vi "Stop Editor.vi"(8 "error in (no error)":errorcluster, 11 "Editor Handler in":refnum<class "Image Editor Handler.lvclass">) -> (0 "error out":errorcluster, 3 "Editor Handler out":refnum<class "Image Editor Handler.lvclass">)   [LabVIEW 2017, in "LV Image Editor Framework.lvlib" / "Image Editor Handler.lvclass"]
uses:
  Image Editor Handler.lvclass
  Image Editor Handler.lvclass/Image Editor Handler.ctl
  Forms/Shape/Shape.lvclass
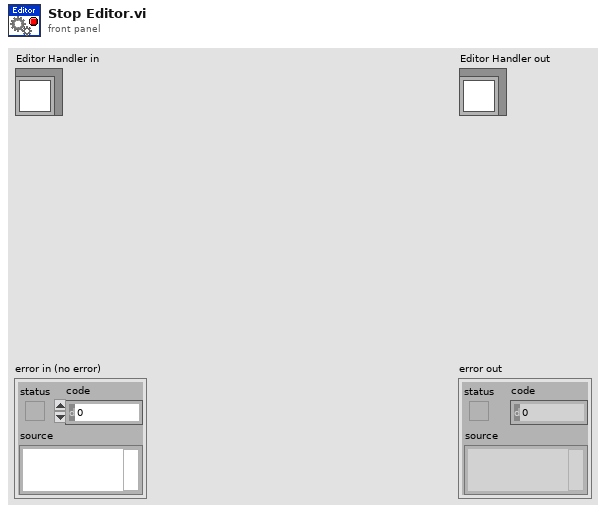
[diagram p1: front panel]
types:
  T1 = typedef "LV Image Editor Framework.lvlib/Image Editor Handler.lvclass/Editor Events.ctl" = cluster{"Stop":refnum<user-event>, "Image Events":cluster{"AddShape":refnum<user-event>, "Paint":refnum<user-event>, "RemoveShape":refnum<user-event>, "RefreshShape ByRef":refnum<user-event>, "ShapePropertyChange":refnum<user-event>, "RemoveShape ByRef":refnum<user-event>}, "RequestShapes":refnum<user-event>, "Custom":refnum<user-event>}
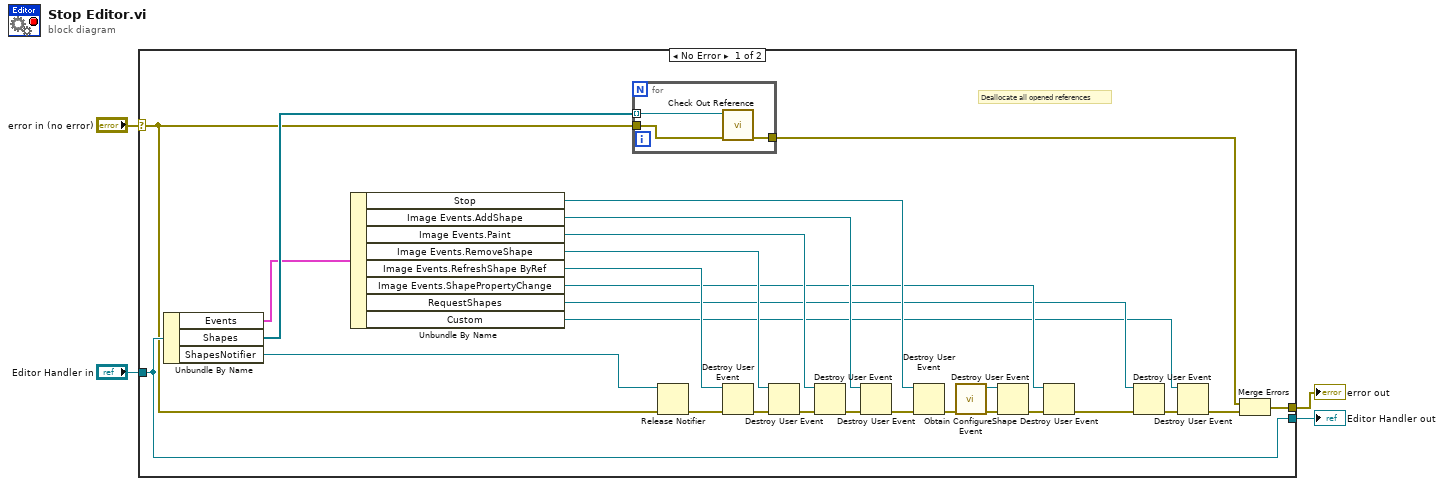
[diagram p0: block diagram]
diagram:
  n1 = case shown="No Error" "error in (no error)" {
    selector: "error in (no error)" -> [w7 w36]
    tunnel: [w17 w36] -> w3
    tunnel: [w31 w35] -> w1
    tunnel: "Editor Handler in" -> [w31 w35]
    frame No Error {
      # "Deallocate all opened references"
      n2 = Unbundle By Name(w31) -> ("Events"=w29:T1, "Shapes"=w30:refnum<data-value>[], "ShapesNotifier"=w13:refnum<notifier>)
      n3 = Unbundle By Name(w29) -> ("Stop"=w24:refnum<user-event>, "Image Events.AddShape"=w25:refnum<user-event>, "Image Events.Paint"=w26:refnum<user-event>, "Image Events.RemoveShape"=w27:refnum<user-event>, "Image Events.RefreshShape ByRef"=w28:refnum<user-event>, "Image Events.ShapePropertyChange"=w16:refnum<user-event>, "RequestShapes"=w15:refnum<user-event>, "Custom"=w14:refnum<user-event>)
      n4 = for {
        tunnel: w30 -> [w34] mode=indexing
        tunnel: [w33] -> w10
        tunnel: w7 -> [w32]
        n5 = call "Check Out Reference.vi"("error in (no error)"=w32, "Shape Reference"=w34) -> ("error out"=w33:errorcluster)  [unwired: 9 in]
      }
      n6 = Release Notifier(notifier=w13, error in (no error)=w7) -> (error out=w6:errorcluster)  [unwired: 1 in, 2 out]
      n7 = Destroy User Event(user event=w28, error in=w6) -> (error out=w23:errorcluster)
      n8 = Destroy User Event(user event=w27, error in=w23) -> (error out=w22:errorcluster)
      n9 = Destroy User Event(user event=w26, error in=w22) -> (error out=w21:errorcluster)
      n10 = Destroy User Event(user event=w25, error in=w21) -> (error out=w9:errorcluster)
      n11 = Destroy User Event(user event=w24, error in=w9) -> (error out=w18:errorcluster)
      n12 = call "Obtain ConfigureShape Event.vi"("error in (no error)"=w18) -> ("error out"=w20:errorcluster, "ShapeChanged Event"=w19:refnum<user-event>)  [unwired: 9 in]
      n13 = Destroy User Event(user event=w19, error in=w20) -> (error out=w11:errorcluster)
      n14 = Destroy User Event(user event=w16, error in=w11) -> (error out=w5:errorcluster)
      n15 = Destroy User Event(user event=w15, error in=w5) -> (error out=w12:errorcluster)
      n16 = Destroy User Event(user event=w14, error in=w12) -> (error out=w8:errorcluster)
      n17 = Merge Errors(w10, w8) -> (w17:errorcluster)
    }
    frame Error {
    }
  }
  "error out" <- w3
  "Editor Handler out" <- w1
